vi "fletcher32.vi"(1 "UPDread out":u8[](array[numeric])) -> (0 "checksum":u8[](array[numeric]))   [LabVIEW 2017]
panel:
  out "s1":u32
  out "s0":u32
  out "uint16 taken":u32[](array[numeric])
  out "reformat":u8[][](array[numeric])
  # "vételkor a checksumot az udpreaden belül a reshape elõtt lehet kivenni"
  # "[2^15;2^16-1]"
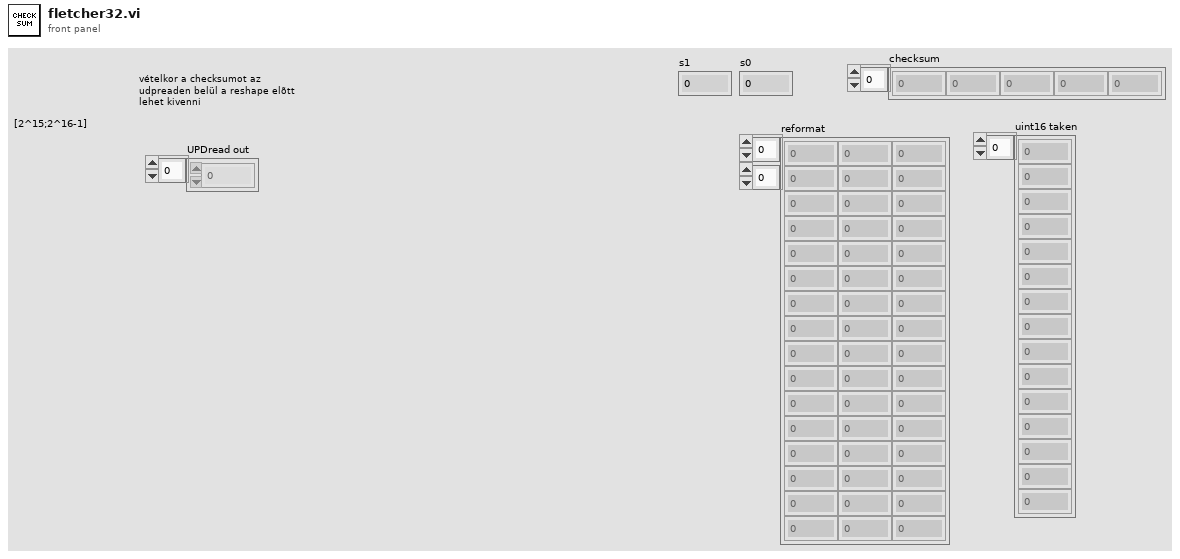
[diagram p1: front panel]
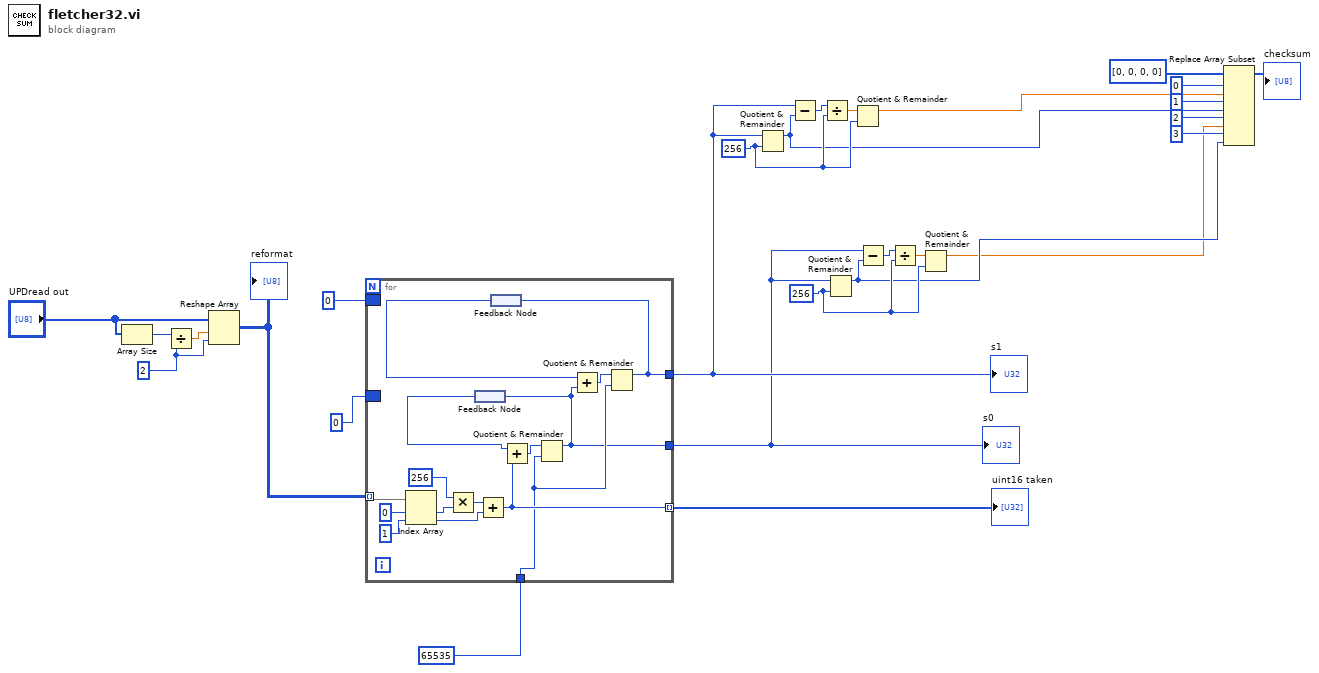
[diagram p0: block diagram]
diagram:
  w9 = u32 256 ("y")
  w12 = u32 256 ("y")
  w25 = 2 ("y")
  n1 = Array Size(array="UPDread out") -> (size(s)=w27:i32)
  n2 = Divide(x=w27, y=w25) -> (x/y=w26:dbl)
  n3 = Reshape Array("UPDread out", w26, w25) -> (w24:u8[][])
  "reformat" <- w24
  n4 = for {
    tunnel: w24 -> [w42] mode=indexing
    tunnel: [w31] -> w15
    tunnel: [w29] -> w7
    tunnel: [w35] -> w23 mode=indexing
    tunnel: 65535 ("divisor") -> [w32]
    border: 0 ("init s1") -> [_]
    border: 0 ("init s0") -> [_]
    n5 = Index Array(array=w42, index #1=0 ("index"), index #2=1 ("index")) -> (element #1=w39:u8, element #2=w36:u8)
    n6 = Multiply(x=u32 256, y=w39) -> (x*y=w37:u32)
    n7 = feedback #1() -> (w28:u32)
    n8 = Add(x=w37, y=w36) -> (x+y=w35:u32)
    n9 = feedback #2() -> (w30:u32)
    n10 = Add(x=w28, y=w35) -> (x+y=w34:u32)
    n11 = Quotient & Remainder(x=w34, y=w32) -> (x-y*floor(x/y)=w29:u32)  [unwired: 1 out]
    n12 = feedback-in #1(w29) -> ()
    n13 = Add(x=w30, y=w29) -> (x+y=w33:u32)
    n14 = Quotient & Remainder(x=w33, y=w32) -> (x-y*floor(x/y)=w31:u32)  [unwired: 1 out]
    n15 = feedback-in #2(w31) -> ()
  }
  "uint16 taken" <- w23
  "s0" <- w7
  "s1" <- w15
  n16 = Quotient & Remainder(x=w15, y=w12) -> (x-y*floor(x/y)=w4:u32)  [unwired: 1 out]
  n17 = Subtract(x=w15, y=w4) -> (x-y=w13:u32)
  n18 = Divide(x=w13, y=w12) -> (x/y=w14:dbl)
  n19 = Quotient & Remainder(x=w7, y=w9) -> (x-y*floor(x/y)=w6:u32)  [unwired: 1 out]
  n20 = Quotient & Remainder(x=w14, y=w12) -> (x-y*floor(x/y)=w8:dbl)  [unwired: 1 out]
  n21 = Subtract(x=w7, y=w6) -> (x-y=w10:u32)
  n22 = Divide(x=w10, y=w9) -> (x/y=w11:dbl)
  n23 = Quotient & Remainder(x=w11, y=w9) -> (x-y*floor(x/y)=w5:dbl)  [unwired: 1 out]
  n24 = Replace Array Subset(array=u8[] [0, 0, 0, 0], new element #1=w8, index #1=0 ("index"), new element #2=w4, index #2=1 ("index"), new element #3=w5, index #3=2 ("index"), new element #4=w6, index #4=3 ("index")) -> (→"checksum":u8[])
